vi "TestExec.Result, Overwrite Numeric Data.vi"(7 "Module Q Name":string, 8 "error in":errorcluster, 10 "Numeric Data":T1[](array[typedef]) {"Status" items=["LOG", "PASS", "FAIL", "ERROR"]}, 11 "Q In":refnum<queue>) -> (0 "error out":errorcluster)   [LabVIEW 2018]
uses:
  <vilib>/KATE/Queues/Q.Element.ctl
  Results/Result.Numeric.ctl
  Results/Result.Limit Type.ctl
  Results/Result.Measurement and Attribute Item Status.ctl
  <vilib>/KATE/Queues/Queue Utils.lvlib
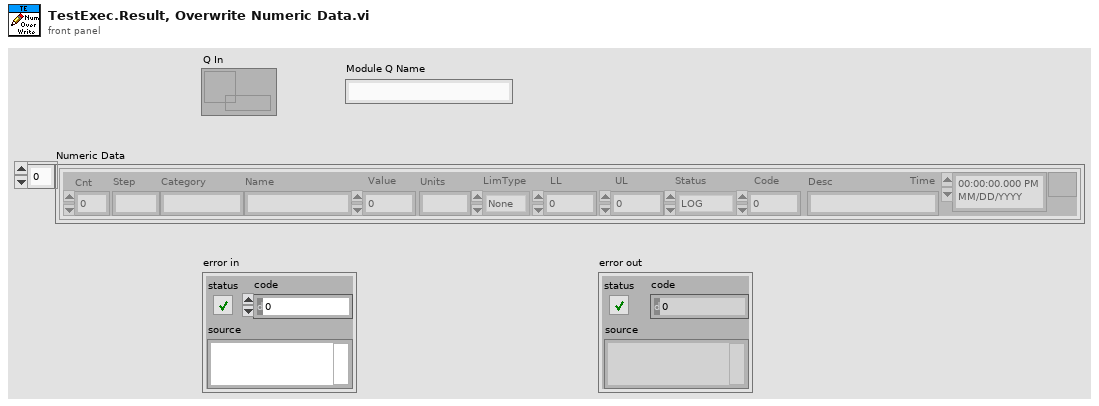
[diagram p1: front panel]
types:
  T1 = typedef "Result.Numeric.ctl" = cluster{"Cnt":i32, "Step":string, "Category":string, "Name":string, "Value":dbl, "Units":string, "LimType":T2, "LL":dbl, "UL":dbl, "Status":T3, "Code":i32, "Desc":string, "Time":timestamp}
  T2 = typedef "Result.Limit Type.ctl" = enum16{"None", "EQ", "NE", "GT", "LT", "GE", "LE", "GTLT", "GELE", "GELT", "GTLE", "LTGT", "LEGE", "LEGT", "LTGE"}
  T3 = typedef "Result.Measurement and Attribute Item Status.ctl" = i32
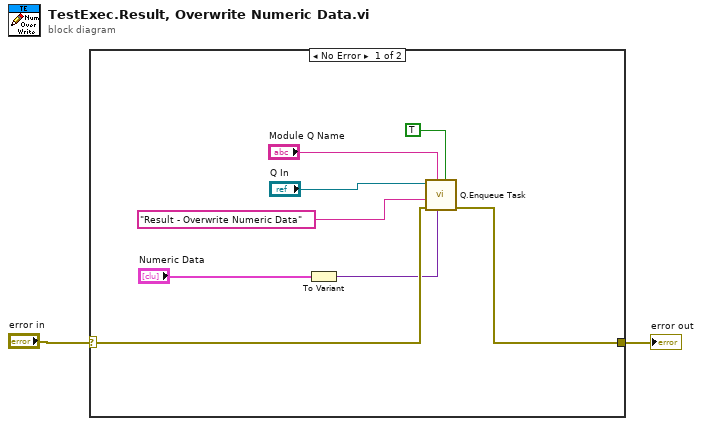
[diagram p0: block diagram]
diagram:
  n1 = case shown="No Error" "error in" {
    selector: "error in" -> [w7 w11]
    tunnel: [w8 w11] -> w1
    frame No Error {
      n2 = To Variant(anything="Numeric Data") -> (Variant=w6:variant)
      n3 = call <vilib>:"Q.Enqueue Task.vi"("Top of Q"=TRUE, "Data1"=w6, "Q Name"="Module Q Name", "Error In"=w7, "Task Name"="Result - Overwrite Numeric Data" ("Cmd"), "Q In"="Q In") -> ("error out"=w8:errorcluster)  [unwired: 4 in, 1 out]
    }
    frame Error {
    }
  }
  "error out" <- w1
